vi "Demo.vi"() -> ()   [LabVIEW 2009]
uses:
  MVCAMSDK.dll
panel:
  in  "Stop 2":bool
  out "Video 2":T1(plugin-control)
  in  "显示相机参数面板 2":bool
  in  "拍照 2":bool
  in  "激活预览 2":bool
  in  "要写入相机2的字符串(32字节)":string
  in  "写入自定义数据 2":bool
  out "从相机2中读出的字符串(32字节)":string
  in  "读取自定义数据 2":bool
  out "Video":T1(plugin-control)
  in  "读取自定义数据":bool
  out "从相机1中读出的字符串(32字节)":string
  in  "写入自定义数据":bool
  in  "要写入相机1的字符串(32字节)":string
  in  "拍照":bool
  in  "显示相机参数面板":bool
  in  "Stop":bool
  in  "激活预览":bool
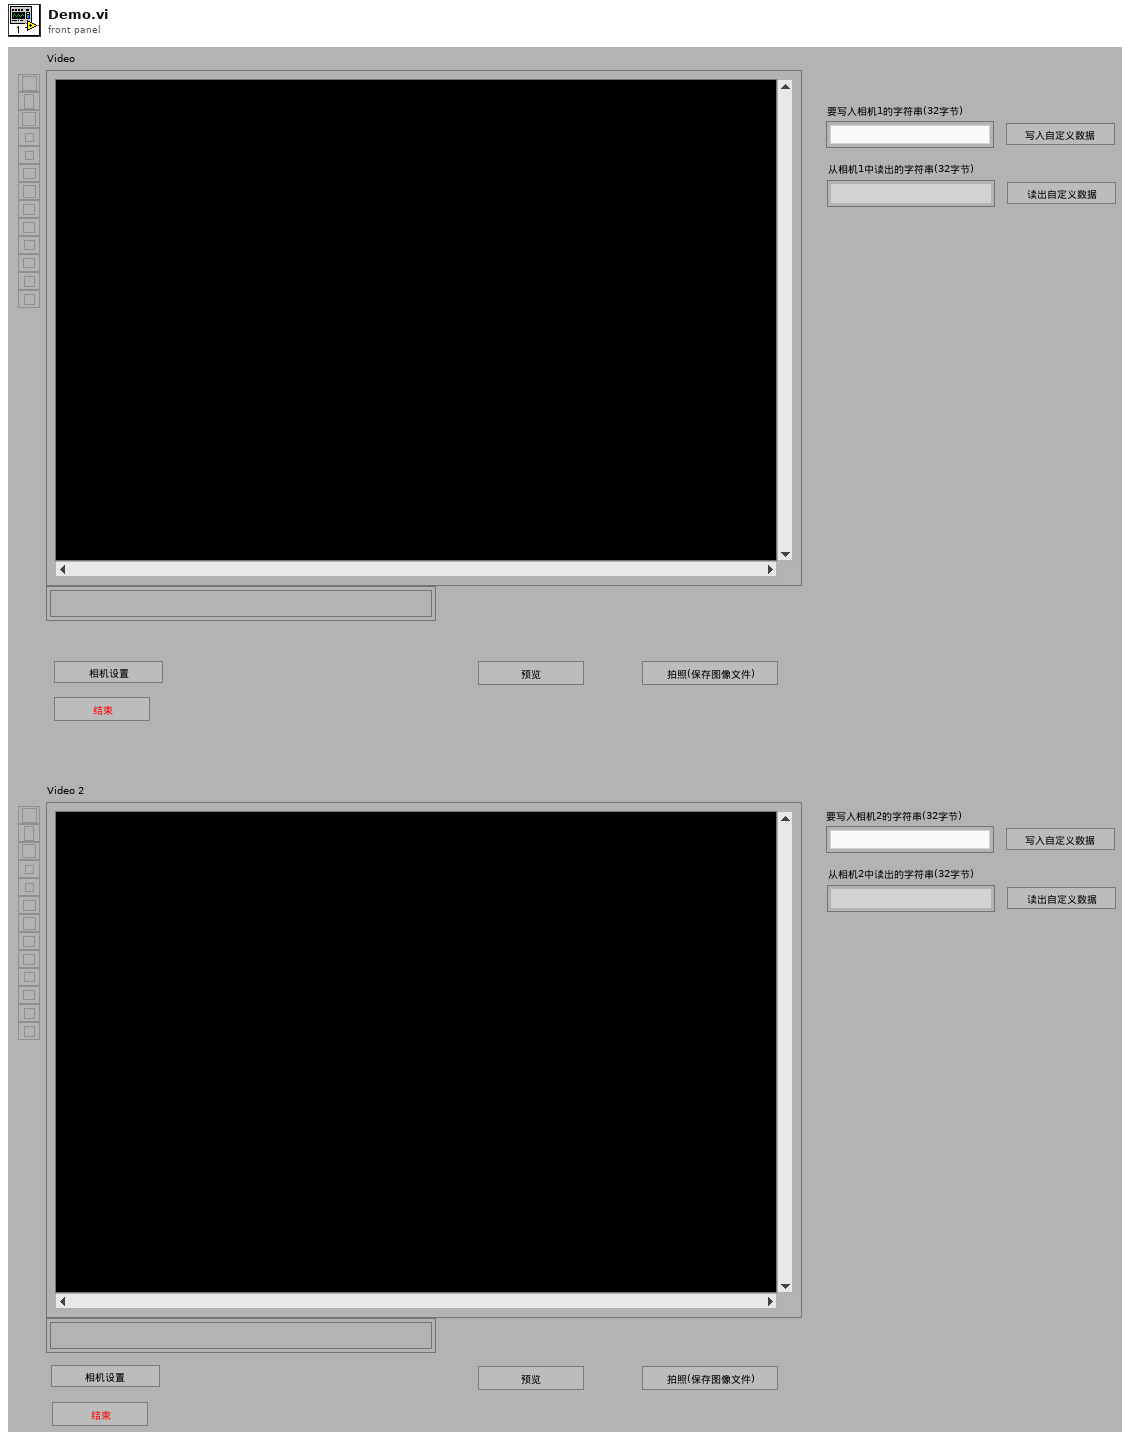
[diagram p1: front panel]
types:
  T1 = typedef "IMAQ Image.ctl" = refnum<image>
  T2 = typedef "Image Type" = u32
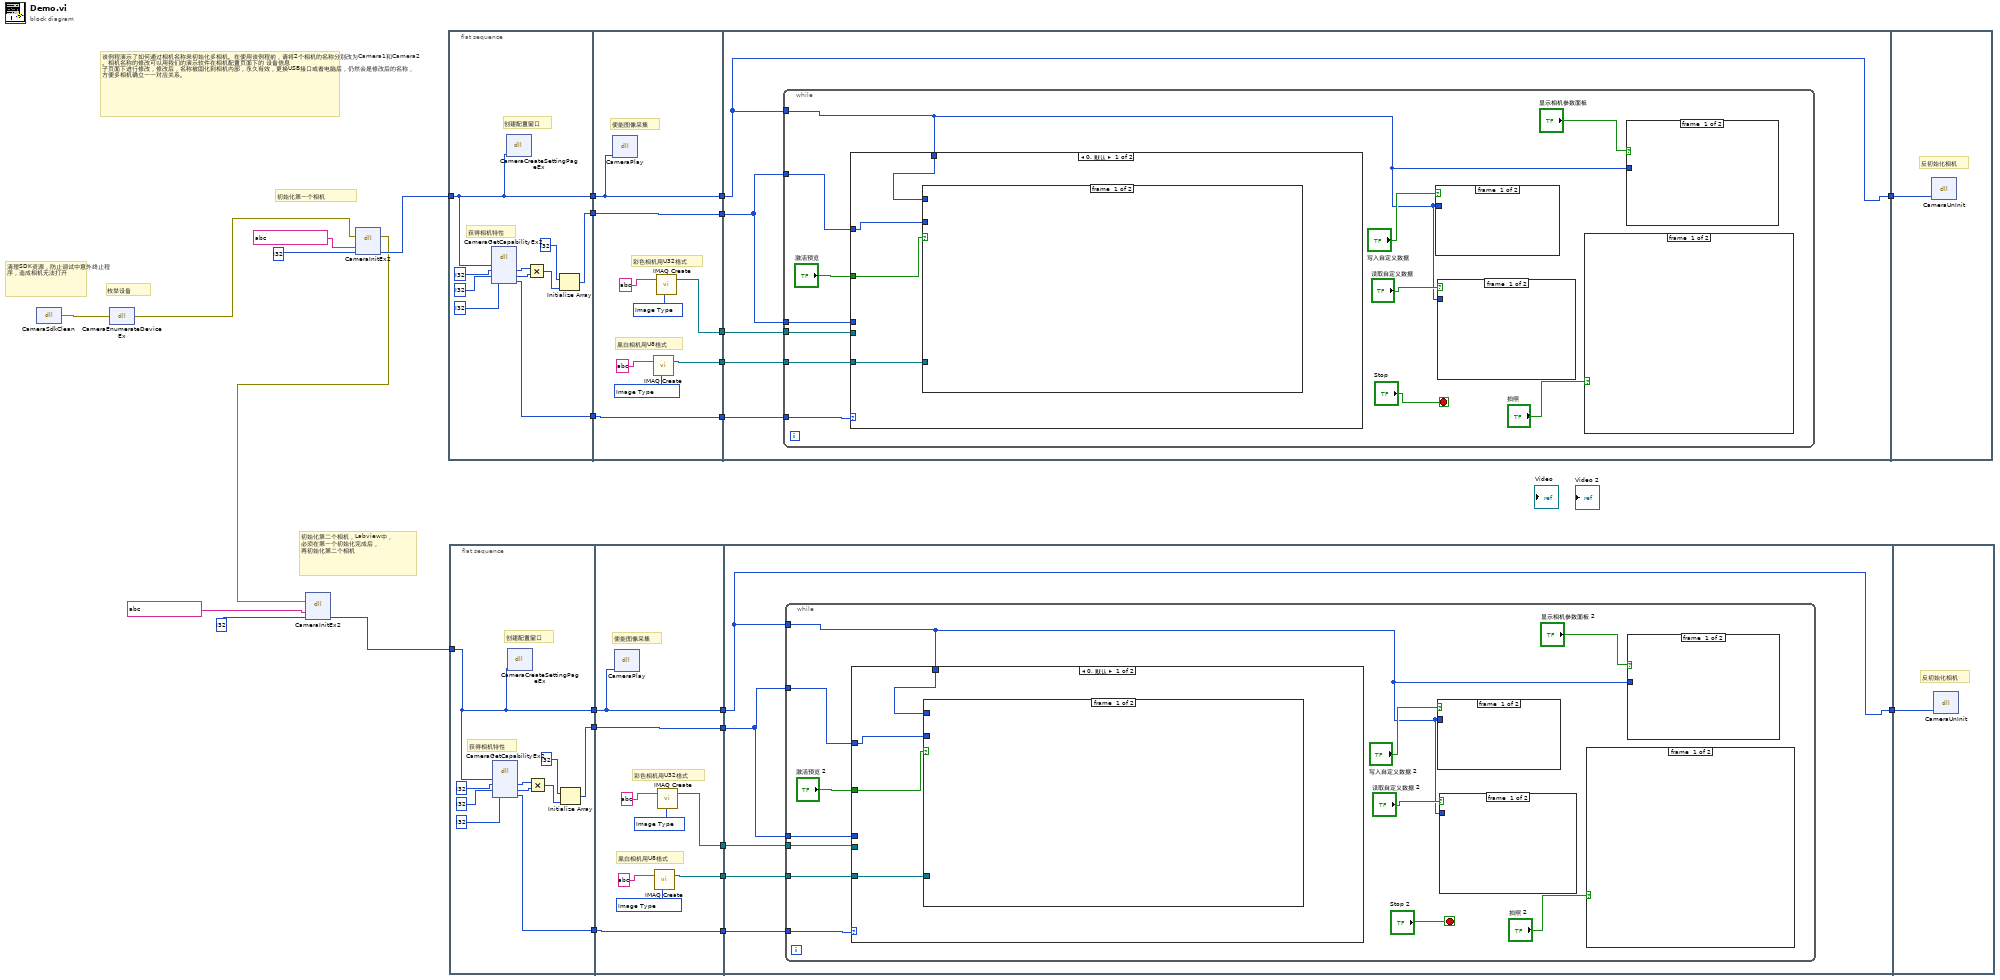
[diagram p0: block diagram]
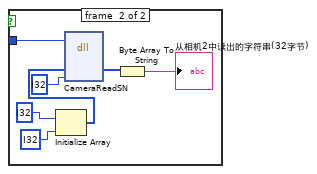
[diagram p2: hidden frame]
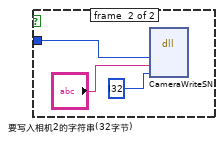
[diagram p3: hidden frame]
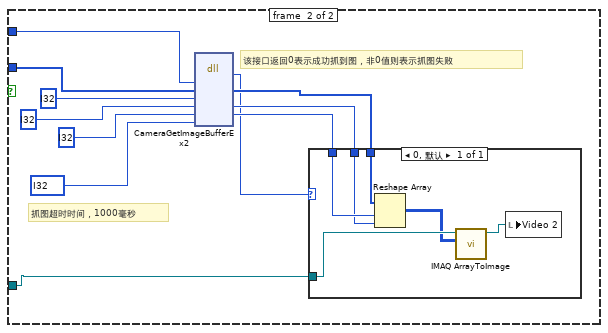
[diagram p4: hidden frame]
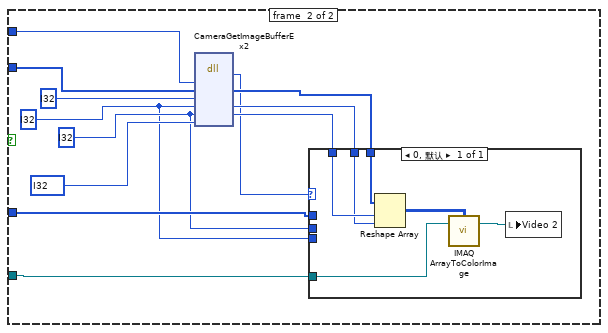
[diagram p6: hidden frame]
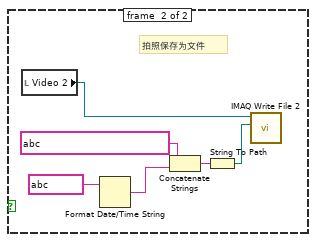
[diagram p7: hidden frame]
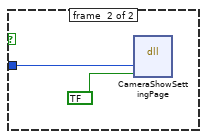
[diagram p8: hidden frame]
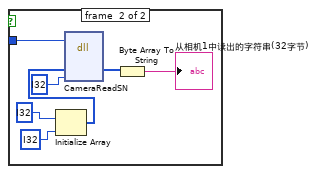
[diagram p9: hidden frame]
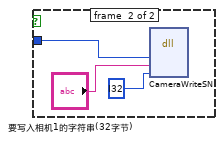
[diagram p10: hidden frame]
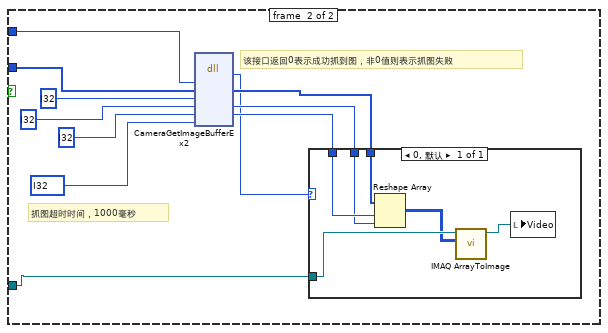
[diagram p11: hidden frame]
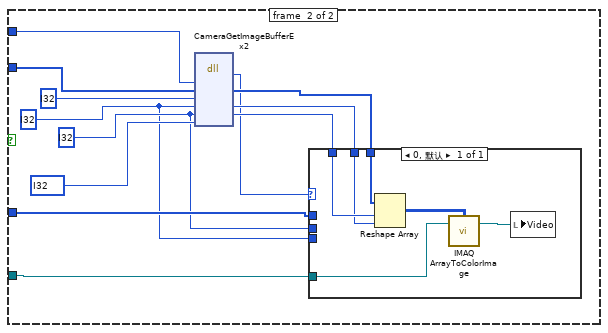
[diagram p13: hidden frame]
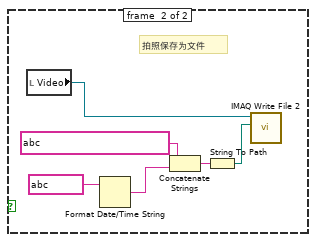
[diagram p14: hidden frame]
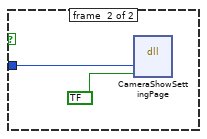
[diagram p15: hidden frame]
diagram:
  # "该例程演示了如何通过相机名称来初始化多相机。在使用该例程前，请将2个相机的名称分别改为Camera1和Camera2。相机名称的修改可以用我们的演示软件在相机配置页面下的 设备信息 子页面下进行修改，修改后，名称被固化到相机内部，永久有效，更换USB接口或者电脑后，仍然会是修改后的名称，方便多相机确立一一对应关系。"
  # "枚举设备"
  # "清理SDK资源，防止调试中意外终止程序，造成相机无法打开"
  # "初始化第一个相机"
  # "初始化第二个相机，Labview中，\n必须在第一个初始化完成后，\n再初始化第二个相机"
  n1 = dll-call lib="MVCAMSDK.dll" fn="CameraSdkClean"() -> (error out=w3:errorcluster)  [unwired: 4 in, 1 out]
  n2 = dll-call lib="MVCAMSDK.dll" fn="CameraEnumerateDeviceEx"(error in=w3) -> (error out=w2:errorcluster)  [unwired: 3 in, 1 out]
  n3 = dll-call lib="MVCAMSDK.dll" fn="CameraInitEx2"(error in=w2, "相机名称"=string ?, "相机句柄"=i32 ?) -> (error out=w1:errorcluster, "相机句柄"=w5:i32)  [unwired: 4 in, 1 out]
  n4 = dll-call lib="MVCAMSDK.dll" fn="CameraInitEx2"(error in=w1, "相机名称"=string ?, "相机句柄"=i32 ?) -> ("相机句柄"=w4:i32)  [unwired: 4 in, 2 out]
  n5 = flat-sequence {
    tunnel: [w28] -> w24
    tunnel: [w35] -> w23
    tunnel: [w29] -> w21
    tunnel: w5 -> [w28]
    tunnel: w24 -> [w46]
    tunnel: [w46] -> w27
    tunnel: [w43] -> w25
    tunnel: w23 -> [w42]
    tunnel: [w42] -> w22
    tunnel: w21 -> [w41]
    tunnel: [w41] -> w20
    tunnel: [w38] -> w19
    tunnel: w27 -> [w49]
    tunnel: [w49] -> w26
    tunnel: w25 -> [w51]
    tunnel: w22 -> [w47]
    tunnel: w20 -> [w50]
    tunnel: w19 -> [w48]
    tunnel: w26 -> [w126]
    frame #0 {
      # "获得相机特性"
      # "创建配置窗口"
      n6 = dll-call lib="MVCAMSDK.dll" fn="CameraGetCapabilityEx2"("相机句柄"=w28, "图像最大宽度"=i32 ?, "图像最大高度"=i32 ?, "是否是彩色相机(返回0:黑白;1:彩色)"=i32 ?) -> ("图像最大宽度"=w31:i32, "图像最大高度"=w30:i32, "是否是彩色相机(返回0:黑白;1:彩色)"=w29:i32)  [unwired: 5 in, 2 out]
      n7 = dll-call lib="MVCAMSDK.dll" fn="CameraCreateSettingPageEx"("相机句柄"=w28) -> ()  [unwired: 5 in, 2 out]
      n8 = Multiply(x=w31, y=w30) -> (x*y=w36:i32)
      n9 = Initialize Array(i32 ?, w36) -> (w35:i32[])
    }
    frame #1 {
      w40 = T2 ? items=["Grayscale (U8)", "Grayscale (I16)", "Grayscale (SGL)", "Complex (CSG)", "RGB (U32)", "HSL (U32)", "RGB (U64)", "Grayscale (U16)"] ("Image Type")
      w45 = T2 ? items=["Grayscale (U8)", "Grayscale (I16)", "Grayscale (SGL)", "Complex (CSG)", "RGB (U32)", "HSL (U32)", "RGB (U64)", "Grayscale (U16)"] ("Image Type")
      # "黑白相机用U8格式"
      # "彩色相机用U32格式"
      # "使能图像采集"
      n10 = dll-call lib="MVCAMSDK.dll" fn="CameraPlay"("相机句柄"=w46) -> ()  [unwired: 5 in, 2 out]
      n11 = call "IMAQ Create"("Image Name"=string ?, "Image Type"=w40) -> ("New Image"=w38:T1)  [unwired: 3 in, 1 out]
      n12 = call "IMAQ Create"("Image Name"=string ?, "Image Type"=w45) -> ("New Image"=w43:T1)  [unwired: 3 in, 1 out]
    }
    frame #2 {
      n13 = while {
        tunnel: w49 -> [w53]
        tunnel: w51 -> [w60]
        tunnel: w47 -> [w61]
        tunnel: w50 -> [w59]
        tunnel: w48 -> [w57]
        tunnel: w47 -> [w56]
        stop <- "Stop" stop-if-true
        n14 = case shown="0, 默认" w59 {
          tunnel: w61 -> [w75 w99]
          tunnel: w60 -> [_ w96]
          tunnel: w53 -> [w76 w98]
          tunnel: "激活预览" -> [w74 w97]
          tunnel: w57 -> [w77 _]
          tunnel: w56 -> [_ w95]
          frame #0 {
            n15 = case shown="真" w74 {
              tunnel: w76 -> [_ w88]
              tunnel: w75 -> [_ w79]
              tunnel: w77 -> [_ w78]
              frame #0 {
              }
              frame #1 {
                # "该接口返回0表示成功抓到图，非0值则表示抓图失败"
                # "抓图超时时间，1000毫秒"
                n16 = dll-call lib="MVCAMSDK.dll" fn="CameraGetImageBufferEx2"("相机句柄"=w88, "图像数据缓冲区"=w79, "图像输出格式(0:8位灰度;1:24位彩色;2:32位彩色)"=i32 ?, "图像宽度"=i32 ?, "图像高度"=i32 ?, "抓图超时时间(毫秒)"=i32 ?) -> ("返回类型"=w80:i32, "图像数据缓冲区"=w83:u8[], "图像宽度"=w81:i32, "图像高度"=w82:i32)  [unwired: 6 in, 2 out]
                n17 = case shown="0, 默认" w80 {
                  tunnel: w83 -> [w94]
                  tunnel: w78 -> [w91]
                  tunnel: w82 -> [w93]
                  tunnel: w81 -> [w92]
                  frame 0, 默认 {
                    n18 = Reshape Array(w94, w93, w92) -> (w90:u8[][])
                    n19 = call "IMAQ ArrayToImage"("Image Pixels (U8)"=w90, "Image"=w91) -> ("Image Out"=w89:T1)  [unwired: 8 in, 1 out]
                    n20 = local write "Video"(w89) -> ()
                  }
                }
              }
            }
          }
          frame #1 {
            n21 = case shown="真" w97 {
              tunnel: w98 -> [_ w111]
              tunnel: w96 -> [_ w104]
              tunnel: w99 -> [_ w103]
              tunnel: w95 -> [_ w102]
              frame #0 {
              }
              frame #1 {
                w100 = i32 ?
                w101 = i32 ?
                n22 = dll-call lib="MVCAMSDK.dll" fn="CameraGetImageBufferEx2"("相机句柄"=w111, "图像数据缓冲区"=w103, "图像输出格式(0:8位灰度;1:24位彩色;2:32位彩色)"=i32 ?, "图像宽度"=w100, "图像高度"=w101, "抓图超时时间(毫秒)"=i32 ?) -> ("返回类型"=w105:i32, "图像数据缓冲区"=w108:u32[], "图像宽度"=w106:i32, "图像高度"=w107:i32)  [unwired: 6 in, 2 out]
                n23 = case shown="0, 默认" w105 {
                  tunnel: w108 -> [w115]
                  tunnel: w104 -> [w114]
                  tunnel: w107 -> [w113]
                  tunnel: w106 -> [w112]
                  tunnel: w102 -> [_]
                  tunnel: w101 -> [_]
                  tunnel: w100 -> [_]
                  frame 0, 默认 {
                    n24 = Reshape Array(w115, w113, w112) -> (w116:u32[][])
                    n25 = call "IMAQ ArrayToColorImage"("Image Pixels (U32)"=w116, "Image"=w114) -> ("Image Out"=w117:T1)  [unwired: 3 in, 1 out]
                    n26 = local write "Video"(w117) -> ()
                  }
                }
              }
            }
          }
        }
        n27 = case shown="真" "写入自定义数据" {
          tunnel: w53 -> [_ w73]
          frame #0 {
          }
          frame #1 {
            n28 = dll-call lib="MVCAMSDK.dll" fn="CameraWriteSN"("相机句柄"=w73, "序列号(固定为32个字节)"="要写入相机1的字符串(32字节)", "序列号级别，[0,1,2]对应3级序列号，其中0级为只读，1,2级可写"=i32 ?) -> ()  [unwired: 7 in, 2 out]
          }
        }
        n29 = case shown="真" "读取自定义数据" {
          tunnel: w53 -> [_ w70]
          frame #0 {
          }
          frame #1 {
            n30 = Initialize Array(i32 ?, i32 ?) -> (w67:i32[])
            n31 = dll-call lib="MVCAMSDK.dll" fn="CameraReadSN"("相机句柄"=w70, "序列号"=w67, "序列号级别，[0,1,2],0级为只读，1,2级可写"=i32 ?) -> ("序列号"=w65:u8[])  [unwired: 6 in, 2 out]
            n32 = Byte Array To String(unsigned byte array=w65) -> (string=→"从相机1中读出的字符串(32字节)":string)
          }
        }
        n33 = case shown="真" "拍照" {
          frame #0 {
          }
          frame #1 {
            # "拍照保存为文件"
            n34 = local read "Video"() -> (w118:T1)
            n35 = Format Date/Time String(time format string (%c)=string ?) -> (date/time string=w122:string)  [unwired: 2 in]
            n36 = Concatenate Strings(string ?, w122) -> (w119:string)
            n37 = String To Path(string=w119) -> (path=w121:path)
            n38 = call-poly "IMAQ Write File 2"("File Path"=w121, "Image"=w118) -> ()  [unwired: 8 in, 2 out]
          }
        }
        n39 = case shown="真" "显示相机参数面板" {
          tunnel: w53 -> [_ w125]
          frame #0 {
          }
          frame #1 {
            n40 = dll-call lib="MVCAMSDK.dll" fn="CameraShowSettingPage"("相机句柄"=w125, "状态"=bool ?) -> ()  [unwired: 6 in, 2 out]
          }
        }
      }
    }
    frame #3 {
      # "反初始化相机"
      n41 = dll-call lib="MVCAMSDK.dll" fn="CameraUnInit"("相机句柄"=w126) -> ()  [unwired: 5 in, 2 out]
    }
  }
  n42 = flat-sequence {
    tunnel: [w127] -> w18
    tunnel: [w134] -> w17
    tunnel: [w128] -> w16
    tunnel: w4 -> [w127]
    tunnel: w18 -> [w145]
    tunnel: [w145] -> w15
    tunnel: [w142] -> w14
    tunnel: w17 -> [w141]
    tunnel: [w141] -> w13
    tunnel: w16 -> [w140]
    tunnel: [w140] -> w12
    tunnel: [w137] -> w11
    tunnel: w15 -> [w148]
    tunnel: [w148] -> w10
    tunnel: w14 -> [w150]
    tunnel: w13 -> [w146]
    tunnel: w12 -> [w149]
    tunnel: w11 -> [w147]
    tunnel: w10 -> [w225]
    frame #0 {
      # "获得相机特性"
      # "创建配置窗口"
      n43 = dll-call lib="MVCAMSDK.dll" fn="CameraGetCapabilityEx2"("相机句柄"=w127, "图像最大宽度"=i32 ?, "图像最大高度"=i32 ?, "是否是彩色相机(返回0:黑白;1:彩色)"=i32 ?) -> ("图像最大宽度"=w130:i32, "图像最大高度"=w129:i32, "是否是彩色相机(返回0:黑白;1:彩色)"=w128:i32)  [unwired: 5 in, 2 out]
      n44 = dll-call lib="MVCAMSDK.dll" fn="CameraCreateSettingPageEx"("相机句柄"=w127) -> ()  [unwired: 5 in, 2 out]
      n45 = Multiply(x=w130, y=w129) -> (x*y=w135:i32)
      n46 = Initialize Array(i32 ?, w135) -> (w134:i32[])
    }
    frame #1 {
      w139 = T2 ? items=["Grayscale (U8)", "Grayscale (I16)", "Grayscale (SGL)", "Complex (CSG)", "RGB (U32)", "HSL (U32)", "RGB (U64)", "Grayscale (U16)"] ("Image Type")
      w144 = T2 ? items=["Grayscale (U8)", "Grayscale (I16)", "Grayscale (SGL)", "Complex (CSG)", "RGB (U32)", "HSL (U32)", "RGB (U64)", "Grayscale (U16)"] ("Image Type")
      # "黑白相机用U8格式"
      # "彩色相机用U32格式"
      # "使能图像采集"
      n47 = dll-call lib="MVCAMSDK.dll" fn="CameraPlay"("相机句柄"=w145) -> ()  [unwired: 5 in, 2 out]
      n48 = call "IMAQ Create"("Image Name"=string ?, "Image Type"=w139) -> ("New Image"=w137:T1)  [unwired: 3 in, 1 out]
      n49 = call "IMAQ Create"("Image Name"=string ?, "Image Type"=w144) -> ("New Image"=w142:T1)  [unwired: 3 in, 1 out]
    }
    frame #2 {
      n50 = while {
        tunnel: w148 -> [w152]
        tunnel: w150 -> [w159]
        tunnel: w146 -> [w160]
        tunnel: w149 -> [w158]
        tunnel: w147 -> [w156]
        tunnel: w146 -> [w155]
        stop <- "Stop 2" stop-if-true
        n51 = case shown="0, 默认" w158 {
          tunnel: w160 -> [w174 w198]
          tunnel: w159 -> [_ w195]
          tunnel: w152 -> [w175 w197]
          tunnel: "激活预览 2" -> [w173 w196]
          tunnel: w156 -> [w176 _]
          tunnel: w155 -> [_ w194]
          frame #0 {
            n52 = case shown="真" w173 {
              tunnel: w175 -> [_ w187]
              tunnel: w174 -> [_ w178]
              tunnel: w176 -> [_ w177]
              frame #0 {
              }
              frame #1 {
                # "该接口返回0表示成功抓到图，非0值则表示抓图失败"
                # "抓图超时时间，1000毫秒"
                n53 = dll-call lib="MVCAMSDK.dll" fn="CameraGetImageBufferEx2"("相机句柄"=w187, "图像数据缓冲区"=w178, "图像输出格式(0:8位灰度;1:24位彩色;2:32位彩色)"=i32 ?, "图像宽度"=i32 ?, "图像高度"=i32 ?, "抓图超时时间(毫秒)"=i32 ?) -> ("返回类型"=w179:i32, "图像数据缓冲区"=w182:u8[], "图像宽度"=w180:i32, "图像高度"=w181:i32)  [unwired: 6 in, 2 out]
                n54 = case shown="0, 默认" w179 {
                  tunnel: w182 -> [w193]
                  tunnel: w177 -> [w190]
                  tunnel: w181 -> [w192]
                  tunnel: w180 -> [w191]
                  frame 0, 默认 {
                    n55 = Reshape Array(w193, w192, w191) -> (w189:u8[][])
                    n56 = call "IMAQ ArrayToImage"("Image Pixels (U8)"=w189, "Image"=w190) -> ("Image Out"=w188:T1)  [unwired: 8 in, 1 out]
                    n57 = local write "Video 2"(w188) -> ()
                  }
                }
              }
            }
          }
          frame #1 {
            n58 = case shown="真" w196 {
              tunnel: w197 -> [_ w210]
              tunnel: w195 -> [_ w203]
              tunnel: w198 -> [_ w202]
              tunnel: w194 -> [_ w201]
              frame #0 {
              }
              frame #1 {
                w199 = i32 ?
                w200 = i32 ?
                n59 = dll-call lib="MVCAMSDK.dll" fn="CameraGetImageBufferEx2"("相机句柄"=w210, "图像数据缓冲区"=w202, "图像输出格式(0:8位灰度;1:24位彩色;2:32位彩色)"=i32 ?, "图像宽度"=w199, "图像高度"=w200, "抓图超时时间(毫秒)"=i32 ?) -> ("返回类型"=w204:i32, "图像数据缓冲区"=w207:u32[], "图像宽度"=w205:i32, "图像高度"=w206:i32)  [unwired: 6 in, 2 out]
                n60 = case shown="0, 默认" w204 {
                  tunnel: w207 -> [w214]
                  tunnel: w203 -> [w213]
                  tunnel: w206 -> [w212]
                  tunnel: w205 -> [w211]
                  tunnel: w201 -> [_]
                  tunnel: w200 -> [_]
                  tunnel: w199 -> [_]
                  frame 0, 默认 {
                    n61 = Reshape Array(w214, w212, w211) -> (w215:u32[][])
                    n62 = call "IMAQ ArrayToColorImage"("Image Pixels (U32)"=w215, "Image"=w213) -> ("Image Out"=w216:T1)  [unwired: 3 in, 1 out]
                    n63 = local write "Video 2"(w216) -> ()
                  }
                }
              }
            }
          }
        }
        n64 = case shown="真" "写入自定义数据 2" {
          tunnel: w152 -> [_ w172]
          frame #0 {
          }
          frame #1 {
            n65 = dll-call lib="MVCAMSDK.dll" fn="CameraWriteSN"("相机句柄"=w172, "序列号(固定为32个字节)"="要写入相机2的字符串(32字节)", "序列号级别，[0,1,2]对应3级序列号，其中0级为只读，1,2级可写"=i32 ?) -> ()  [unwired: 7 in, 2 out]
          }
        }
        n66 = case shown="真" "读取自定义数据 2" {
          tunnel: w152 -> [_ w169]
          frame #0 {
          }
          frame #1 {
            n67 = Initialize Array(i32 ?, i32 ?) -> (w166:i32[])
            n68 = dll-call lib="MVCAMSDK.dll" fn="CameraReadSN"("相机句柄"=w169, "序列号"=w166, "序列号级别，[0,1,2],0级为只读，1,2级可写"=i32 ?) -> ("序列号"=w164:u8[])  [unwired: 6 in, 2 out]
            n69 = Byte Array To String(unsigned byte array=w164) -> (string=→"从相机2中读出的字符串(32字节)":string)
          }
        }
        n70 = case shown="真" "拍照 2" {
          frame #0 {
          }
          frame #1 {
            # "拍照保存为文件"
            n71 = local read "Video 2"() -> (w217:T1)
            n72 = Format Date/Time String(time format string (%c)=string ?) -> (date/time string=w221:string)  [unwired: 2 in]
            n73 = Concatenate Strings(string ?, w221) -> (w218:string)
            n74 = String To Path(string=w218) -> (path=w220:path)
            n75 = call-poly "IMAQ Write File 2"("File Path"=w220, "Image"=w217) -> ()  [unwired: 8 in, 2 out]
          }
        }
        n76 = case shown="真" "显示相机参数面板 2" {
          tunnel: w152 -> [_ w224]
          frame #0 {
          }
          frame #1 {
            n77 = dll-call lib="MVCAMSDK.dll" fn="CameraShowSettingPage"("相机句柄"=w224, "状态"=bool ?) -> ()  [unwired: 6 in, 2 out]
          }
        }
      }
    }
    frame #3 {
      # "反初始化相机"
      n78 = dll-call lib="MVCAMSDK.dll" fn="CameraUnInit"("相机句柄"=w225) -> ()  [unwired: 5 in, 2 out]
    }
  }
